vi "Untitled 2.vi"() -> ()   [LabVIEW 2020]
uses:
  NAI5330A_TypeDefs.llb/NAI5330A_ModeSelector.ctl
panel:
  in  "Pict Ring":T1
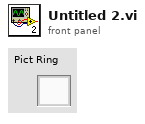
[diagram p1: front panel]
types:
  T1 = typedef "NAI5330A_ModeSelector.ctl" = u16
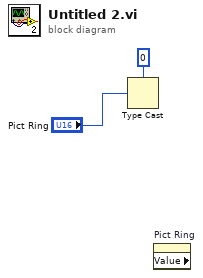
[diagram p0: block diagram]
diagram:
  n1 = Type Cast(type=u16 0, x="Pict Ring") -> ()  [unwired: 1 out]
  n2 = property on="Pict Ring" class="Ring (strict)" props=["Value"]() -> ()  [unwired: 2 in, 3 out]
